vi "PlugIn_Backpack.vi"(9 "queueName":string="PV_script", 10 "Console":string) -> ()   [LabVIEW 2022 SP3]
panel:
  in  "stop":bool
  out "Spike":string
  out "Dongle":string
  in  "Send to backpack":string
  in  "Send":bool
  in  "Clear":bool
  in  "Ctrl C":bool
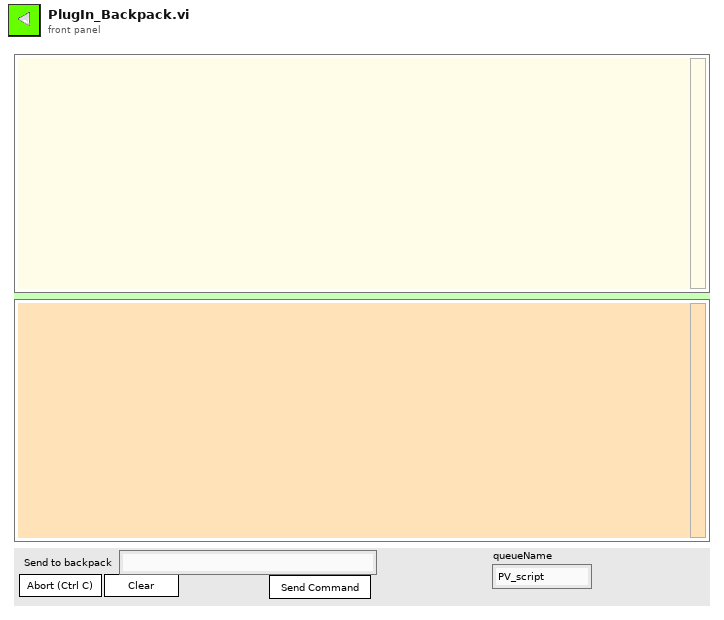
[diagram p1: front panel]
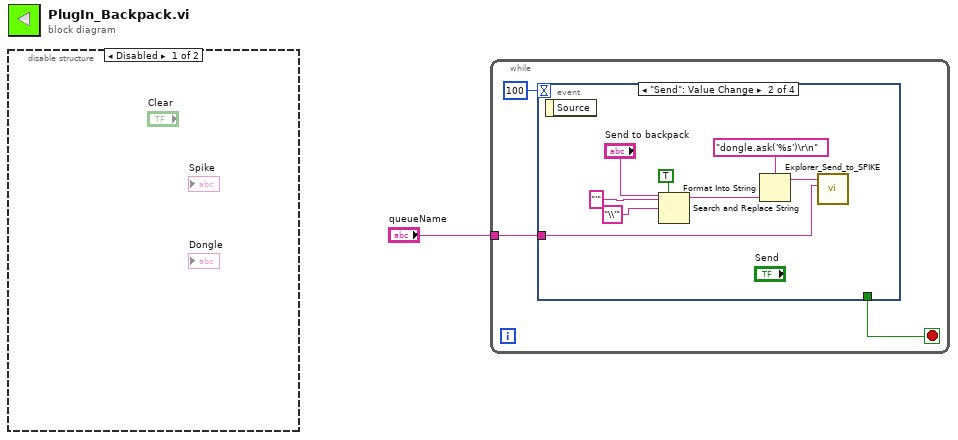
[diagram p0: block diagram]
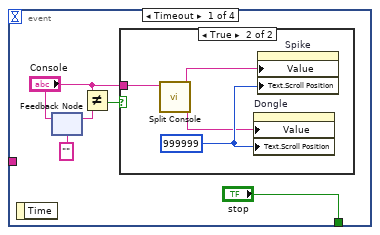
[diagram p2: hidden frame]
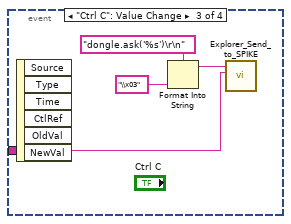
[diagram p4: hidden frame]
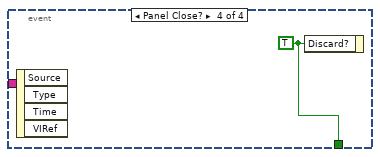
[diagram p5: hidden frame]
diagram:
  n1 = disable-structure shown="Disabled" {
    frame Disabled {
    }
    frame Enabled {
    }
  }
  n2 = while {
    tunnel: "queueName" -> [w2]
    stop <- w4 stop-if-true
    n3 = event shown="[1] \"Send\": Value Change" {
      selector: _ -> [_ _ _ _]
      dyn-events: _ -> [_ _ _ _]
      timeout: 100 -> [_ _ _ _]
      tunnel: ["stop" _ _ w26] -> w4
      tunnel: w2 -> [_ w14 w22 _]
      event Timeout {
        n4 = event-data() -> ()  [unwired: 1 in, 1 out]
        n5 = feedback-in #1("Console") -> ()
        n6 = feedback #1("" ("Console")) -> (w8:string)
        n7 = Not Equal?(x="Console", y=w8) -> (x != y?=w5:bool)
        n8 = case shown="True" w5 {
          tunnel: "Console" -> [_ w13]
          frame False {
          }
          frame True {
            w12 = u32 999999 ("Text.Selection:End")
            n9 = call "Split Console.vi"("Console"=w13) -> ("Dongle"=w10:string, "Spike"=w11:string)  [unwired: 9 in]
            n10 = property on="Dongle" class="Str"("Value"=w10, "Text.Scroll Position"=w12) -> ()  [unwired: 2 in, 2 out]
            n11 = property on="Spike" class="Str"("Value"=w11, "Text.Scroll Position"=w12) -> ()  [unwired: 2 in, 2 out]
          }
        }
      }
      event "Send": Value Change {
        n12 = event-data() -> ()  [unwired: 1 in, 1 out]
        n13 = Search and Replace String(replace all?=TRUE ("replace all? (F)"), input string="Send to backpack", search string="'" ("string"), replace string="\\'" ("string")) -> (result string=w17:string)  [unwired: 4 in, 3 out]
        n14 = Format Into String(format string="dongle.ask('%s')\r\n" ("string"), w17) -> (resulting string=w21:string)  [unwired: 2 in, 1 out]
        n15 = call "Explorer_Send_to_SPIKE.vi"("queueName"=w14, "python"=w21) -> ()  [unwired: 9 in, 1 out]
      }
      event "Ctrl C": Value Change {
        n16 = event-data() -> ()  [unwired: 1 in, 6 out]
        n17 = Format Into String(format string="dongle.ask('%s')\r\n" ("string"), "\\x03" ("Send to backpack 2")) -> (resulting string=w24:string)  [unwired: 2 in, 1 out]
        n18 = call "Explorer_Send_to_SPIKE.vi"("queueName"=w22, "python"=w24) -> ()  [unwired: 9 in, 1 out]
      }
      event Panel Close? {
        w26 = TRUE ("Discard?")
        n19 = event-data() -> ()  [unwired: 1 in, 4 out]
        n20 = event-data("Discard?"=w26) -> ()  [unwired: 1 in, 1 out]
      }
    }
  }
